vi "SubSystems.vi"(8 "error in":errorcluster) -> ()   [LabVIEW 2017]
doc: "This VI calls the various robot subsystems that will then run in parallel. New subSystems will automatlically script code to make the call."
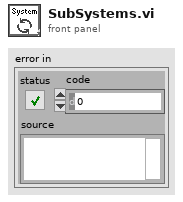
[diagram p1: front panel]
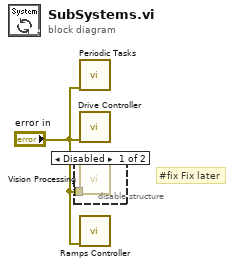
[diagram p0: block diagram]
diagram:
  # "#fix Fix later"
  n1 = disable-structure shown="Disabled" {
    disable-tunnel: "error in" -> [w2 _]
    frame Disabled {
      n2 = call "Vision Processing.vi"("error in (no error)"=w2) -> ()  [unwired: 7 in]
    }
    frame Enabled {
    }
  }
  n3 = call "Periodic Tasks.vi"("error in"="error in") -> ()  [unwired: 1 in, 10 out]
  n4 = call "Drive Controller.vi"("error in"="error in") -> ()  [unwired: 11 in]
  n5 = call "Ramps Controller.vi"("error in"="error in") -> ()  [unwired: 11 in]
